vi "参数.vi"() -> ()   [LabVIEW 2018]
panel:
  in  "LOG":bool
  in  "选项卡控件":T1(tab)
  in  "轮盘关到开终点":dbl=10.0 caption="操作力终点" format="%.2f"
  in  "轮盘关到开起点":dbl=10.0 caption="操作力起点" format="%.2f"
  in  "轮盘关到开锁起点":dbl=10.0 caption="锁止力起点" format="%.2f"
  in  "轮盘关到开锁终点":dbl=10.0 caption="锁止力终点" format="%.2f"
  in  "轮盘关到开锁系数+":sgl=10.0 caption="锁止力系数+" format="%.2f"
  in  "轮盘关到开锁系数x":sgl=10.0 caption="锁止力系数x" format="%.2f"
  in  "轮盘关到开锁上限":sgl=10.0 caption="锁止力上限" format="%.2f"
  in  "轮盘关到开锁下限":sgl=10.0 caption="锁止力下限" format="%.2f"
  in  "轮盘关到开系数":sgl=10.0 caption="操作力系数" format="%.2f"
  in  "轮盘关到开曲线点数":dbl=10.0 caption="曲线点数"
  in  "轮盘关到开上限":sgl=10.0 caption="操作力上限" format="%.2f"
  in  "轮盘关到开下限":sgl=10.0 caption="操作力下限" format="%.2f"
  in  "轮盘关到开Y轴上限":dbl=10.0 caption="Y轴上限" format="%.1f"
  in  "轮盘关到开Y轴下限":dbl=10.0 caption="Y轴下限" format="%.1f"
  in  "轮盘开到关终点":dbl=10.0 caption="操作力终点" format="%.2f"
  in  "轮盘开到关起点":dbl=10.0 caption="操作力起点" format="%.2f"
  in  "轮盘开到关锁起点":dbl=10.0 caption="锁止力起点" format="%.2f"
  in  "轮盘开到关锁终点":dbl=10.0 caption="锁止力终点" format="%.2f"
  in  "轮盘开到关锁系数+":sgl=10.0 caption="锁止力系数+" format="%.2f"
  in  "轮盘开到关锁系数x":sgl=10.0 caption="锁止力系数x" format="%.2f"
  in  "轮盘开到关锁上限":sgl=10.0 caption="锁止力上限" format="%.2f"
  in  "轮盘开到关锁下限":sgl=10.0 caption="锁止力下限" format="%.2f"
  in  "轮盘开到关系数":sgl=10.0 caption="操作力系数" format="%.2f"
  in  "轮盘开到关曲线点数":dbl=10.0 caption="曲线点数"
  in  "轮盘开到关上限":sgl=10.0 caption="操作力上限" format="%.2f"
  in  "轮盘开到关下限":sgl=10.0 caption="操作力下限" format="%.2f"
  in  "轮盘开到关Y轴上限":dbl=10.0 caption="Y轴上限" format="%.1f"
  in  "轮盘开到关Y轴下限":dbl=10.0 caption="Y轴下限" format="%.1f"
  in  "拨钮右到左终点":dbl=10.0 caption="操作力终点" format="%.2f"
  in  "拨钮右到左起点":dbl=10.0 caption="操作力起点" format="%.2f"
  in  "拨钮右到左系数":sgl=10.0 caption="操作力系数" format="%.2f"
  in  "拨钮右到左曲线点数":dbl=10.0 caption="曲线点数"
  in  "拨钮右到左上限":sgl=10.0 caption="操作力上限" format="%.2f"
  in  "拨钮右到左下限":sgl=10.0 caption="操作力下限" format="%.2f"
  in  "拨钮右到左Y轴上限":dbl=10.0 caption="Y轴上限" format="%.1f"
  in  "拨钮右到左Y轴下限":dbl=10.0 caption="Y轴下限" format="%.1f"
  in  "拨钮左到右终点":dbl=10.0 caption="操作力终点" format="%.2f"
  in  "拨钮左到右起点":dbl=10.0 caption="操作力起点" format="%.2f"
  in  "拨钮左到右系数":sgl=10.0 caption="操作力系数" format="%.2f"
  in  "拨钮左到右曲线点数":dbl=10.0 caption="曲线点数"
  in  "拨钮左到右上限":sgl=10.0 caption="操作力上限" format="%.2f"
  in  "拨钮左到右下限":sgl=10.0 caption="操作力下限" format="%.2f"
  in  "拨钮左到右Y轴上限":dbl=10.0 caption="Y轴上限" format="%.1f"
  in  "拨钮左到右Y轴下限":dbl=10.0 caption="Y轴下限" format="%.1f"
  in  "拨钮下到上终点":dbl=10.0 caption="操作力终点" format="%.2f"
  in  "拨钮下到上起点":dbl=10.0 caption="操作力起点" format="%.2f"
  in  "拨钮下到上系数":sgl=10.0 caption="操作力系数" format="%.2f"
  in  "拨钮下到上曲线点数":dbl=10.0 caption="曲线点数"
  in  "拨钮下到上上限":sgl=10.0 caption="操作力上限" format="%.2f"
  in  "拨钮下到上下限":sgl=10.0 caption="操作力下限" format="%.2f"
  in  "拨钮下到上Y轴上限":dbl=10.0 caption="Y轴上限" format="%.1f"
  in  "拨钮下到上Y轴下限":dbl=10.0 caption="Y轴下限" format="%.1f"
  in  "拨钮上到下终点":dbl=10.0 caption="操作力终点" format="%.2f"
  in  "拨钮上到下起点":dbl=10.0 caption="操作力起点" format="%.2f"
  in  "拨钮上到下系数":sgl=10.0 caption="操作力系数" format="%.2f"
  in  "拨钮上到下曲线点数":dbl=10.0 caption="曲线点数"
  in  "拨钮上到下上限":sgl=10.0 caption="操作力上限" format="%.2f"
  in  "拨钮上到下下限":sgl=10.0 caption="操作力下限" format="%.2f"
  in  "拨钮上到下Y轴上限":dbl=10.0 caption="Y轴上限" format="%.1f"
  in  "拨钮上到下Y轴下限":dbl=10.0 caption="Y轴下限" format="%.1f"
  in  "伺服速度":sgl caption="N" format="%.1f"
  in  "气压稳定时间":sgl caption="N" format="%.1f"
  in  "LED电流下限":sgl caption="N" format="%.2f"
  in  "LED电流上限":sgl caption="N" format="%.2f"
  in  "风门开电压下限":sgl caption="N" format="%.2f"
  in  "风门开电压上限":sgl caption="N" format="%.2f"
  in  "风门闭电压下限":sgl caption="N" format="%.2f"
  in  "风门闭电压上限":sgl caption="N" format="%.2f"
  in  "压力下限":sgl caption="N" format="%.1f"
  in  "压力上限":sgl caption="N" format="%.1f"
  in  "泄漏量上限":sgl caption="N" format="%.2f"
  out "有值改变":bool
  in  "停止":bool
  in  "轮盘预压力":sgl caption="N" format="%.1f"
  # "参数设置"
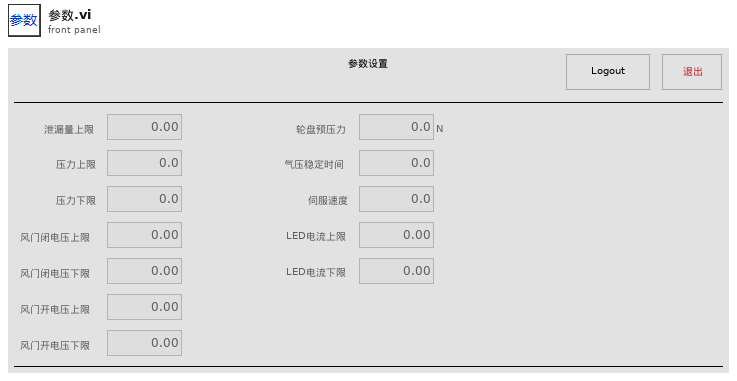
[diagram p1: front panel]
types:
  T1 = enum32{"轮盘关到开", "轮盘开到关", "拨钮右到左", "拨钮左到右", "拨钮下到上", "拨钮上到下"}
  T2 = enum8{"Enabled", "Disabled", "Disabled and Grayed Out"}
  T3 = cluster{"轮盘预压力":sgl, "泄漏量上限":sgl, "压力上限":sgl, "压力下限":sgl, "风门闭电压上限":sgl, "风门闭电压下限":sgl, "风门开电压上限":sgl, "风门开电压下限":sgl, "LED电流上限":sgl, "LED电流下限":sgl, "气压稳定时间":sgl, "伺服速度":sgl}
  T4 = cluster{"选择":enum16{"Fx", "Fy", "Fz", "Mx", "My", "Mz"}, "系数":sgl, "上限":sgl, "下限":sgl, "Ymax":dbl, "Ymin":dbl, "点数":dbl, "锁系数x":sgl, "锁上限":sgl, "锁下限":sgl, "锁系数+":sgl, "起点":dbl, "终点":dbl, "锁起点":dbl, "锁终点":dbl}
  T5 = cluster{"选择":enum16{"Fx", "Fy", "Fz", "Mx", "My", "Mz"}, "系数":sgl, "上限":sgl, "下限":sgl, "Ymax":dbl, "Ymin":dbl, "点数":dbl, "起点":dbl, "终点":dbl}
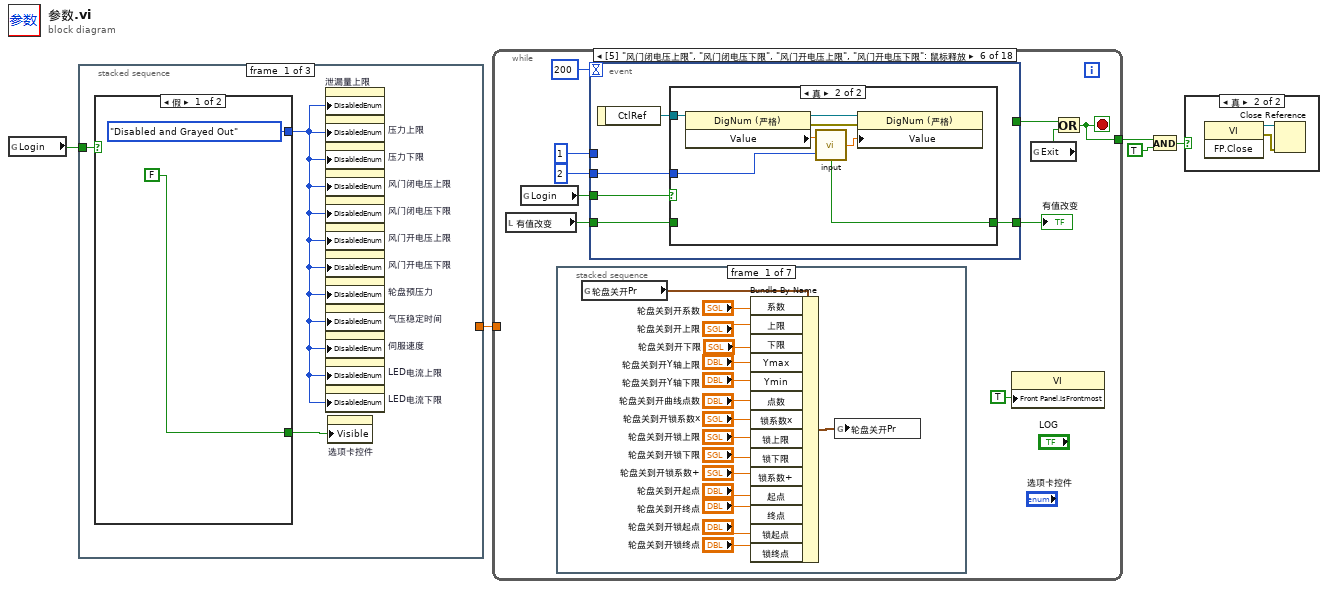
[diagram p0: block diagram]
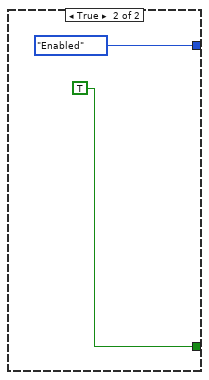
[diagram p2: hidden frame]
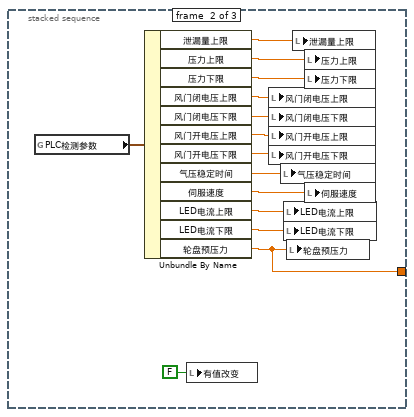
[diagram p3: hidden frame]
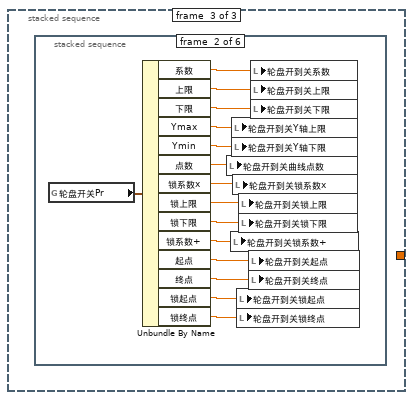
[diagram p4: hidden frame]
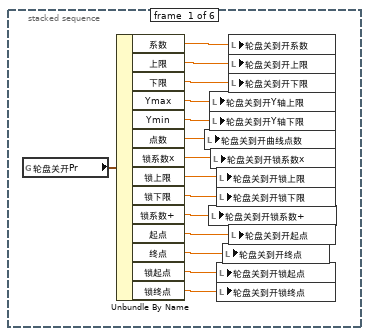
[diagram p5: hidden frame]
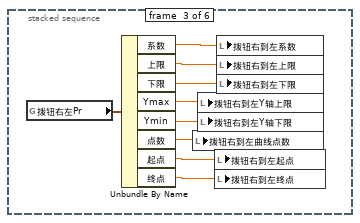
[diagram p6: hidden frame]
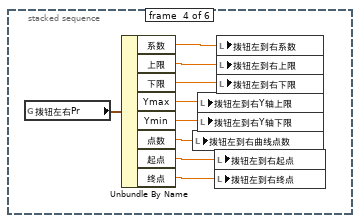
[diagram p7: hidden frame]
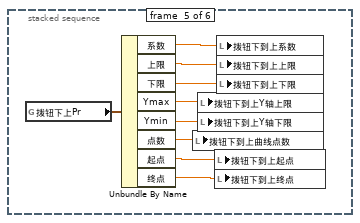
[diagram p8: hidden frame]
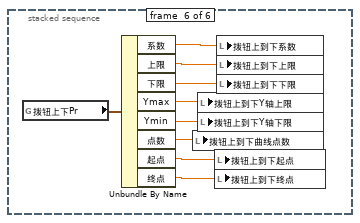
[diagram p9: hidden frame]
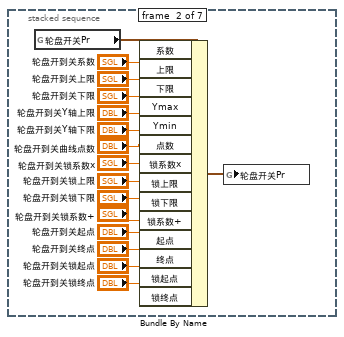
[diagram p11: hidden frame]
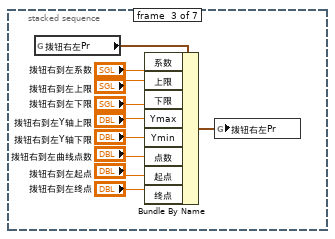
[diagram p12: hidden frame]
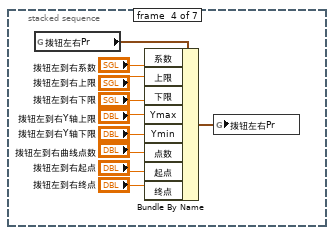
[diagram p13: hidden frame]
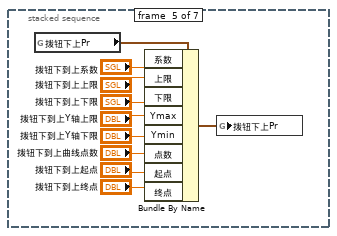
[diagram p14: hidden frame]
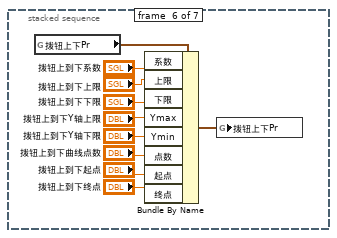
[diagram p15: hidden frame]
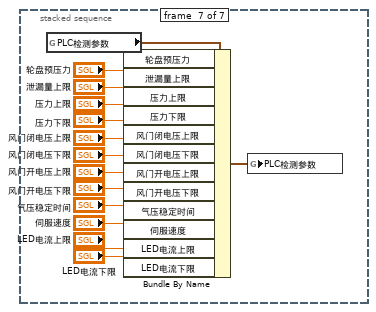
[diagram p16: hidden frame]
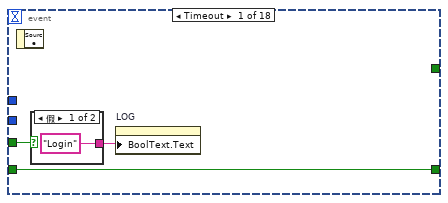
[diagram p17: hidden frame]
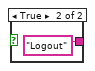
[diagram p18: hidden frame]
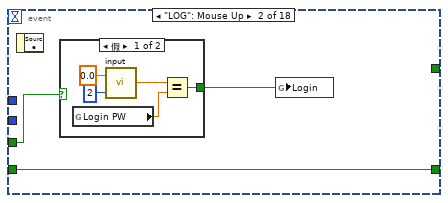
[diagram p19: hidden frame]
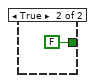
[diagram p20: hidden frame]
diagram:
  n1 = global read "全局 1.vi" "Login"() -> (w1:bool)
  n2 = stacked-sequence {
    tunnel: [_ w13 _] -> w2
    tunnel: w1 -> [w7 _ _]
    frame #0 {
      n3 = case shown="假" w7 {
        tunnel: [T2."Disabled and Grayed Out" ("禁用") T2."Enabled" ("禁用")] -> w8
        tunnel: [FALSE ("可见") TRUE ("可见")] -> w6
        frame False {
        }
        frame True {
        }
      }
      n4 = property on="泄漏量上限" class="DigNum (严格)"("DisabledEnum"=w8) -> ()  [unwired: 2 in, 2 out]
      n5 = property on="压力上限" class="DigNum (严格)"("DisabledEnum"=w8) -> ()  [unwired: 2 in, 2 out]
      n6 = property on="压力下限" class="DigNum (严格)"("DisabledEnum"=w8) -> ()  [unwired: 2 in, 2 out]
      n7 = property on="风门闭电压上限" class="DigNum (严格)"("DisabledEnum"=w8) -> ()  [unwired: 2 in, 2 out]
      n8 = property on="风门闭电压下限" class="DigNum (严格)"("DisabledEnum"=w8) -> ()  [unwired: 2 in, 2 out]
      n9 = property on="风门开电压上限" class="DigNum (严格)"("DisabledEnum"=w8) -> ()  [unwired: 2 in, 2 out]
      n10 = property on="风门开电压下限" class="DigNum (严格)"("DisabledEnum"=w8) -> ()  [unwired: 2 in, 2 out]
      n11 = property on="轮盘预压力" class="DigNum (严格)"("DisabledEnum"=w8) -> ()  [unwired: 2 in, 2 out]
      n12 = property on="气压稳定时间" class="DigNum (严格)"("DisabledEnum"=w8) -> ()  [unwired: 2 in, 2 out]
      n13 = property on="伺服速度" class="DigNum (严格)"("DisabledEnum"=w8) -> ()  [unwired: 2 in, 2 out]
      n14 = property on="LED电流上限" class="DigNum (严格)"("DisabledEnum"=w8) -> ()  [unwired: 2 in, 2 out]
      n15 = property on="LED电流下限" class="DigNum (严格)"("DisabledEnum"=w8) -> ()  [unwired: 2 in, 2 out]
      n16 = property on="选项卡控件" class="TabCtl (严格)"("Visible"=w6) -> ()  [unwired: 2 in, 2 out]
    }
    frame #1 {
      n17 = global read "全局 1.vi" "PLC检测参数"() -> (w15:T3)
      n18 = Unbundle By Name(w15) -> ("泄漏量上限"=w26:sgl, "压力上限"=w25:sgl, "压力下限"=w24:sgl, "风门闭电压上限"=w23:sgl, "风门闭电压下限"=w22:sgl, "风门开电压上限"=w21:sgl, "风门开电压下限"=w20:sgl, "气压稳定时间"=w19:sgl, "伺服速度"=w18:sgl, "LED电流上限"=w17:sgl, "LED电流下限"=w16:sgl, "轮盘预压力"=w13:sgl)
      n19 = local write "有值改变"(FALSE ("有值改变")) -> ()
      n20 = local write "风门闭电压上限"(w23) -> ()
      n21 = local write "风门闭电压下限"(w22) -> ()
      n22 = local write "风门开电压上限"(w21) -> ()
      n23 = local write "风门开电压下限"(w20) -> ()
      n24 = local write "气压稳定时间"(w19) -> ()
      n25 = local write "LED电流上限"(w17) -> ()
      n26 = local write "LED电流下限"(w16) -> ()
      n27 = local write "轮盘预压力"(w13) -> ()
      n28 = local write "泄漏量上限"(w26) -> ()
      n29 = local write "压力上限"(w25) -> ()
      n30 = local write "压力下限"(w24) -> ()
      n31 = local write "伺服速度"(w18) -> ()
    }
    frame #2 {
      n32 = stacked-sequence {
        frame #0 {
          n33 = global read "全局 1.vi" "轮盘关开Pr"() -> (w41:T4)
          n34 = Unbundle By Name(w41) -> ("系数"=w40:sgl, "上限"=w38:sgl, "下限"=w37:sgl, "Ymax"=w36:dbl, "Ymin"=w35:dbl, "点数"=w39:dbl, "锁系数x"=w32:sgl, "锁上限"=w34:sgl, "锁下限"=w33:sgl, "锁系数+"=w31:sgl, "起点"=w30:dbl, "终点"=w29:dbl, "锁起点"=w28:dbl, "锁终点"=w27:dbl)
          n35 = local write "轮盘关到开曲线点数"(w39) -> ()
          n36 = local write "轮盘关到开锁系数+"(w31) -> ()
          n37 = local write "轮盘关到开Y轴上限"(w36) -> ()
          n38 = local write "轮盘关到开Y轴下限"(w35) -> ()
          n39 = local write "轮盘关到开锁系数x"(w32) -> ()
          n40 = local write "轮盘关到开锁上限"(w34) -> ()
          n41 = local write "轮盘关到开锁下限"(w33) -> ()
          n42 = local write "轮盘关到开锁起点"(w28) -> ()
          n43 = local write "轮盘关到开锁终点"(w27) -> ()
          n44 = local write "轮盘关到开终点"(w29) -> ()
          n45 = local write "轮盘关到开系数"(w40) -> ()
          n46 = local write "轮盘关到开上限"(w38) -> ()
          n47 = local write "轮盘关到开下限"(w37) -> ()
          n48 = local write "轮盘关到开起点"(w30) -> ()
        }
        frame #1 {
          n49 = global read "全局 1.vi" "轮盘开关Pr"() -> (w56:T4)
          n50 = Unbundle By Name(w56) -> ("系数"=w55:sgl, "上限"=w53:sgl, "下限"=w52:sgl, "Ymax"=w51:dbl, "Ymin"=w50:dbl, "点数"=w54:dbl, "锁系数x"=w49:sgl, "锁上限"=w48:sgl, "锁下限"=w47:sgl, "锁系数+"=w46:sgl, "起点"=w45:dbl, "终点"=w44:dbl, "锁起点"=w43:dbl, "锁终点"=w42:dbl)
          n51 = local write "轮盘开到关曲线点数"(w54) -> ()
          n52 = local write "轮盘开到关锁系数+"(w46) -> ()
          n53 = local write "轮盘开到关Y轴上限"(w51) -> ()
          n54 = local write "轮盘开到关Y轴下限"(w50) -> ()
          n55 = local write "轮盘开到关锁系数x"(w49) -> ()
          n56 = local write "轮盘开到关锁起点"(w43) -> ()
          n57 = local write "轮盘开到关锁终点"(w42) -> ()
          n58 = local write "轮盘开到关锁上限"(w48) -> ()
          n59 = local write "轮盘开到关锁下限"(w47) -> ()
          n60 = local write "轮盘开到关起点"(w45) -> ()
          n61 = local write "轮盘开到关终点"(w44) -> ()
          n62 = local write "轮盘开到关系数"(w55) -> ()
          n63 = local write "轮盘开到关上限"(w53) -> ()
          n64 = local write "轮盘开到关下限"(w52) -> ()
        }
        frame #2 {
          n65 = global read "全局 1.vi" "拨钮右左Pr"() -> (w65:T5)
          n66 = Unbundle By Name(w65) -> ("系数"=w64:sgl, "上限"=w62:sgl, "下限"=w61:sgl, "Ymax"=w60:dbl, "Ymin"=w59:dbl, "点数"=w63:dbl, "起点"=w58:dbl, "终点"=w57:dbl)
          n67 = local write "拨钮右到左曲线点数"(w63) -> ()
          n68 = local write "拨钮右到左Y轴上限"(w60) -> ()
          n69 = local write "拨钮右到左Y轴下限"(w59) -> ()
          n70 = local write "拨钮右到左起点"(w58) -> ()
          n71 = local write "拨钮右到左终点"(w57) -> ()
          n72 = local write "拨钮右到左系数"(w64) -> ()
          n73 = local write "拨钮右到左上限"(w62) -> ()
          n74 = local write "拨钮右到左下限"(w61) -> ()
        }
        frame #3 {
          n75 = global read "全局 1.vi" "拨钮左右Pr"() -> (w74:T5)
          n76 = Unbundle By Name(w74) -> ("系数"=w73:sgl, "上限"=w71:sgl, "下限"=w70:sgl, "Ymax"=w69:dbl, "Ymin"=w68:dbl, "点数"=w72:dbl, "起点"=w67:dbl, "终点"=w66:dbl)
          n77 = local write "拨钮左到右曲线点数"(w72) -> ()
          n78 = local write "拨钮左到右Y轴上限"(w69) -> ()
          n79 = local write "拨钮左到右Y轴下限"(w68) -> ()
          n80 = local write "拨钮左到右起点"(w67) -> ()
          n81 = local write "拨钮左到右终点"(w66) -> ()
          n82 = local write "拨钮左到右系数"(w73) -> ()
          n83 = local write "拨钮左到右上限"(w71) -> ()
          n84 = local write "拨钮左到右下限"(w70) -> ()
        }
        frame #4 {
          n85 = global read "全局 1.vi" "拨钮下上Pr"() -> (w83:T5)
          n86 = Unbundle By Name(w83) -> ("系数"=w82:sgl, "上限"=w80:sgl, "下限"=w79:sgl, "Ymax"=w78:dbl, "Ymin"=w77:dbl, "点数"=w81:dbl, "起点"=w76:dbl, "终点"=w75:dbl)
          n87 = local write "拨钮下到上曲线点数"(w81) -> ()
          n88 = local write "拨钮下到上Y轴上限"(w78) -> ()
          n89 = local write "拨钮下到上Y轴下限"(w77) -> ()
          n90 = local write "拨钮下到上起点"(w76) -> ()
          n91 = local write "拨钮下到上终点"(w75) -> ()
          n92 = local write "拨钮下到上系数"(w82) -> ()
          n93 = local write "拨钮下到上上限"(w80) -> ()
          n94 = local write "拨钮下到上下限"(w79) -> ()
        }
        frame #5 {
          n95 = global read "全局 1.vi" "拨钮上下Pr"() -> (w92:T5)
          n96 = Unbundle By Name(w92) -> ("系数"=w91:sgl, "上限"=w89:sgl, "下限"=w88:sgl, "Ymax"=w87:dbl, "Ymin"=w86:dbl, "点数"=w90:dbl, "起点"=w84:dbl, "终点"=w85:dbl)
          n97 = local write "拨钮上到下曲线点数"(w90) -> ()
          n98 = local write "拨钮上到下Y轴上限"(w87) -> ()
          n99 = local write "拨钮上到下Y轴下限"(w86) -> ()
          n100 = local write "拨钮上到下起点"(w84) -> ()
          n101 = local write "拨钮上到下终点"(w85) -> ()
          n102 = local write "拨钮上到下系数"(w91) -> ()
          n103 = local write "拨钮上到下上限"(w89) -> ()
          n104 = local write "拨钮上到下下限"(w88) -> ()
        }
      }
    }
  }
  n105 = while {
    tunnel: [w99] -> w4
    tunnel: w2 -> [_]
    stop <- w99 stop-if-true
    n106 = local read "有值改变"() -> (w93:bool)
    n107 = global read "全局 1.vi" "Login"() -> (w94:bool)
    n108 = stacked-sequence {
      frame #0 {
        n109 = global read "全局 1.vi" "轮盘关开Pr"() -> (w104:T4)
        n110 = Bundle By Name(cluster=w104, "系数"="轮盘关到开系数", "上限"="轮盘关到开上限", "下限"="轮盘关到开下限", "Ymax"="轮盘关到开Y轴上限", "Ymin"="轮盘关到开Y轴下限", "点数"="轮盘关到开曲线点数", "锁系数x"="轮盘关到开锁系数x", "锁上限"="轮盘关到开锁上限", "锁下限"="轮盘关到开锁下限", "锁系数+"="轮盘关到开锁系数+", "起点"="轮盘关到开起点", "终点"="轮盘关到开终点", "锁起点"="轮盘关到开锁起点", "锁终点"="轮盘关到开锁终点") -> (w103:T4)
        n111 = global write "全局 1.vi" "轮盘关开Pr"(w103) -> ()
      }
      frame #1 {
        n112 = global read "全局 1.vi" "轮盘开关Pr"() -> (w134:T4)
        n113 = Bundle By Name(cluster=w134, "系数"="轮盘开到关系数", "上限"="轮盘开到关上限", "下限"="轮盘开到关下限", "Ymax"="轮盘开到关Y轴上限", "Ymin"="轮盘开到关Y轴下限", "点数"="轮盘开到关曲线点数", "锁系数x"="轮盘开到关锁系数x", "锁上限"="轮盘开到关锁上限", "锁下限"="轮盘开到关锁下限", "锁系数+"="轮盘开到关锁系数+", "起点"="轮盘开到关起点", "终点"="轮盘开到关终点", "锁起点"="轮盘开到关锁起点", "锁终点"="轮盘开到关锁终点") -> (w133:T4)
        n114 = global write "全局 1.vi" "轮盘开关Pr"(w133) -> ()
      }
      frame #2 {
        n115 = global read "全局 1.vi" "拨钮右左Pr"() -> (w144:T5)
        n116 = Bundle By Name(cluster=w144, "系数"="拨钮右到左系数", "上限"="拨钮右到左上限", "下限"="拨钮右到左下限", "Ymax"="拨钮右到左Y轴上限", "Ymin"="拨钮右到左Y轴下限", "点数"="拨钮右到左曲线点数", "起点"="拨钮右到左起点", "终点"="拨钮右到左终点") -> (w143:T5)
        n117 = global write "全局 1.vi" "拨钮右左Pr"(w143) -> ()
      }
      frame #3 {
        n118 = global read "全局 1.vi" "拨钮左右Pr"() -> (w154:T5)
        n119 = Bundle By Name(cluster=w154, "系数"="拨钮左到右系数", "上限"="拨钮左到右上限", "下限"="拨钮左到右下限", "Ymax"="拨钮左到右Y轴上限", "Ymin"="拨钮左到右Y轴下限", "点数"="拨钮左到右曲线点数", "起点"="拨钮左到右起点", "终点"="拨钮左到右终点") -> (w153:T5)
        n120 = global write "全局 1.vi" "拨钮左右Pr"(w153) -> ()
      }
      frame #4 {
        n121 = global read "全局 1.vi" "拨钮下上Pr"() -> (w164:T5)
        n122 = Bundle By Name(cluster=w164, "系数"="拨钮下到上系数", "上限"="拨钮下到上上限", "下限"="拨钮下到上下限", "Ymax"="拨钮下到上Y轴上限", "Ymin"="拨钮下到上Y轴下限", "点数"="拨钮下到上曲线点数", "起点"="拨钮下到上起点", "终点"="拨钮下到上终点") -> (w163:T5)
        n123 = global write "全局 1.vi" "拨钮下上Pr"(w163) -> ()
      }
      frame #5 {
        n124 = global read "全局 1.vi" "拨钮上下Pr"() -> (w174:T5)
        n125 = Bundle By Name(cluster=w174, "系数"="拨钮上到下系数", "上限"="拨钮上到下上限", "下限"="拨钮上到下下限", "Ymax"="拨钮上到下Y轴上限", "Ymin"="拨钮上到下Y轴下限", "点数"="拨钮上到下曲线点数", "起点"="拨钮上到下起点", "终点"="拨钮上到下终点") -> (w173:T5)
        n126 = global write "全局 1.vi" "拨钮上下Pr"(w173) -> ()
      }
      frame #6 {
        n127 = global read "全局 1.vi" "PLC检测参数"() -> (w175:T3)
        n128 = Bundle By Name(cluster=w175, "轮盘预压力"="轮盘预压力", "泄漏量上限"="泄漏量上限", "压力上限"="压力上限", "压力下限"="压力下限", "风门闭电压上限"="风门闭电压上限", "风门闭电压下限"="风门闭电压下限", "风门开电压上限"="风门开电压上限", "风门开电压下限"="风门开电压下限", "气压稳定时间"="气压稳定时间", "伺服速度"="伺服速度", "LED电流上限"="LED电流上限", "LED电流下限"="LED电流下限") -> (w188:T3)
        n129 = global write "全局 1.vi" "PLC检测参数"(w188) -> ()
      }
    }
    n130 = event shown="[5] \"风门闭电压上限\", \"风门闭电压下限\", \"风门开电压上限\", \"风门开电压下限\": 鼠标释放" {
      selector: _ -> [_ _ _ _ _ _ _ _ _ _ _ _ _ _ _ _ _ _]
      dyn-events: _ -> [_ _ _ _ _ _ _ _ _ _ _ _ _ _ _ _ _ _]
      timeout: 200 -> [_ _ _ _ _ _ _ _ _ _ _ _ _ _ _ _ _ _]
      tunnel: [_ _ "停止" _ _ _ _ _ _ _ _ _ _ _ _ _ _ _] -> w98
      tunnel: 1 -> [_ _ _ _ w223 _ _ w262 w275 w288 _ _ _ _ _ w334 w341 _]
      tunnel: 2 -> [_ _ _ w210 _ w236 w246 _ _ _ w298 w307 w314 w321 w328 _ _ _]
      tunnel: [w189 w194 w203 w207 w222 w235 w249 w261 w274 w287 w300 w306 w313 w320 w327 w335 w342 w349] -> w95
      tunnel: w94 -> [w191 w195 _ w209 w220 w234 w248 w260 w273 w286 _ _ _ _ _ _ _ _]
      tunnel: w93 -> [w189 w194 w203 w208 w221 w233 w247 w259 w272 w285 _ _ _ _ _ _ _ _]
      event Timeout {
        n131 = event-data() -> ()  [unwired: 1 in, 1 out]
        n132 = case shown="假" w191 {
          tunnel: ["Login" "Logout"] -> w190
          frame False {
          }
          frame True {
          }
        }
        n133 = property on="LOG" class="Bool"("BoolText.Text"=w190) -> ()  [unwired: 2 in, 2 out]
      }
      event "LOG": Mouse Up {
        n134 = event-data() -> ()  [unwired: 1 in, 1 out]
        n135 = case shown="假" w195 {
          tunnel: [w197 FALSE] -> w196
          frame False {
            n136 = global read "全局 1.vi" "Login PW"() -> (w198:dbl)
            n137 = call "input.vi"("位数(2)"=2, "in"=0.0) -> ("out"=w199:dbl)  [unwired: 1 out]
            n138 = Equal?(x=w199, y=w198) -> (x = y?=w197:bool)
          }
          frame True {
          }
        }
        n139 = global write "全局 1.vi" "Login"(w196) -> ()
      }
      event "停止": Value Change {
        n140 = event-data() -> ()  [unwired: 1 in, 1 out]
        n141 = global read "全局 1.vi" "ini文件"() -> (w204:path)
        n142 = case shown="真" w203 {
          tunnel: w204 -> [_ w206]
          frame False {
          }
          frame True {
            n143 = call "WriteIni.vi"("configuration file path"=w206) -> ()  [unwired: 1 in]
          }
        }
      }
      event "泄漏量上限": Mouse Up {
        n144 = event-data() -> ("CtlRef"=w211:refnum<vi>)  [unwired: 1 in]
        n145 = case shown="假" w209 {
          tunnel: w211 -> [_ w219]
          tunnel: w210 -> [_ w217]
          tunnel: w208 -> [w212 _]
          tunnel: [w212 w213] -> w207
          frame False {
          }
          frame True {
            n146 = property class="DigNum (严格)"(reference=w219) -> (reference out=w216:refnum<vi>, error out=w215:errorcluster, "Value"=w218:sgl)  [unwired: 1 in]
            n147 = call "input.vi"("位数(2)"=w217, "in"=w218) -> ("out"=w214:dbl, "值改变?"=w213:bool)
            n148 = property class="DigNum (严格)"(reference=w216, error in=w215, "Value"=w214) -> ()  [unwired: 2 out]
          }
        }
      }
      event "压力上限", "压力下限": Mouse Up {
        n149 = event-data() -> ("CtlRef"=w224:refnum<vi>)  [unwired: 1 in]
        n150 = case shown="真" w220 {
          tunnel: w224 -> [_ w232]
          tunnel: w223 -> [_ w230]
          tunnel: [w225 w229] -> w222
          tunnel: w221 -> [w225 _]
          frame False {
          }
          frame True {
            n151 = property class="DigNum (严格)"(reference=w232) -> (reference out=w228:refnum<vi>, error out=w227:errorcluster, "Value"=w231:sgl)  [unwired: 1 in]
            n152 = call "input.vi"("位数(2)"=w230, "in"=w231) -> ("out"=w226:dbl, "值改变?"=w229:bool)
            n153 = property class="DigNum (严格)"(reference=w228, error in=w227, "Value"=w226) -> ()  [unwired: 2 out]
          }
        }
      }
      event "风门闭电压上限", "风门闭电压下限", "风门开电压上限", "风门开电压下限": Mouse Up {
        n154 = event-data() -> ("CtlRef"=w237:refnum<vi>)  [unwired: 1 in]
        n155 = case shown="真" w234 {
          tunnel: w237 -> [_ w245]
          tunnel: w236 -> [_ w243]
          tunnel: [w238 w242] -> w235
          tunnel: w233 -> [w238 _]
          frame False {
          }
          frame True {
            n156 = property class="DigNum (严格)"(reference=w245) -> (reference out=w241:refnum<vi>, error out=w240:errorcluster, "Value"=w244:sgl)  [unwired: 1 in]
            n157 = call "input.vi"("位数(2)"=w243, "in"=w244) -> ("out"=w239:dbl, "值改变?"=w242:bool)
            n158 = property class="DigNum (严格)"(reference=w241, error in=w240, "Value"=w239) -> ()  [unwired: 2 out]
          }
        }
      }
      event "LED电流上限", "LED电流下限": Mouse Up {
        n159 = event-data() -> ("CtlRef"=w250:refnum<vi>)  [unwired: 1 in]
        n160 = case shown="真" w248 {
          tunnel: w250 -> [_ w258]
          tunnel: w246 -> [_ w256]
          tunnel: [w251 w255] -> w249
          tunnel: w247 -> [w251 _]
          frame False {
          }
          frame True {
            n161 = property class="DigNum (严格)"(reference=w258) -> (reference out=w254:refnum<vi>, error out=w253:errorcluster, "Value"=w257:sgl)  [unwired: 1 in]
            n162 = call "input.vi"("位数(2)"=w256, "in"=w257) -> ("out"=w252:dbl, "值改变?"=w255:bool)
            n163 = property class="DigNum (严格)"(reference=w254, error in=w253, "Value"=w252) -> ()  [unwired: 2 out]
          }
        }
      }
      event "气压稳定时间": Mouse Up {
        n164 = event-data() -> ("CtlRef"=w263:refnum<vi>)  [unwired: 1 in]
        n165 = case shown="真" w260 {
          tunnel: w263 -> [_ w271]
          tunnel: w262 -> [_ w269]
          tunnel: [w264 w268] -> w261
          tunnel: w259 -> [w264 _]
          frame False {
          }
          frame True {
            n166 = property class="DigNum (严格)"(reference=w271) -> (reference out=w267:refnum<vi>, error out=w266:errorcluster, "Value"=w270:sgl)  [unwired: 1 in]
            n167 = call "input.vi"("位数(2)"=w269, "in"=w270) -> ("out"=w265:dbl, "值改变?"=w268:bool)
            n168 = property class="DigNum (严格)"(reference=w267, error in=w266, "Value"=w265) -> ()  [unwired: 2 out]
          }
        }
      }
      event "伺服速度": Mouse Up {
        n169 = event-data() -> ("CtlRef"=w276:refnum<vi>)  [unwired: 1 in]
        n170 = case shown="假" w273 {
          tunnel: w276 -> [_ w284]
          tunnel: w275 -> [_ w282]
          tunnel: [w277 w281] -> w274
          tunnel: w272 -> [w277 _]
          frame False {
          }
          frame True {
            n171 = property class="DigNum (严格)"(reference=w284) -> (reference out=w279:refnum<vi>, error out=w278:errorcluster, "Value"=w283:sgl)  [unwired: 1 in]
            n172 = call "input.vi"("位数(2)"=w282, "in"=w283) -> ("out"=w280:dbl, "值改变?"=w281:bool)
            n173 = property class="DigNum (严格)"(reference=w279, error in=w278, "Value"=w280) -> ()  [unwired: 2 out]
          }
        }
      }
      event "轮盘预压力": Mouse Up {
        n174 = event-data() -> ("CtlRef"=w289:refnum<vi>)  [unwired: 1 in]
        n175 = case shown="真" w286 {
          tunnel: w289 -> [_ w297]
          tunnel: w288 -> [_ w295]
          tunnel: [w290 w294] -> w287
          tunnel: w285 -> [w290 _]
          frame False {
          }
          frame True {
            n176 = property class="DigNum (严格)"(reference=w297) -> (reference out=w293:refnum<vi>, error out=w292:errorcluster, "Value"=w296:sgl)  [unwired: 1 in]
            n177 = call "input.vi"("位数(2)"=w295, "in"=w296) -> ("out"=w291:dbl, "值改变?"=w294:bool)
            n178 = property class="DigNum (严格)"(reference=w293, error in=w292, "Value"=w291) -> ()  [unwired: 2 out]
          }
        }
      }
      event "拨钮上到下系数", "拨钮下到上系数", "拨钮左到右系数", "拨钮右到左系数", "轮盘开到关系数", "轮盘关到开系数", "轮盘关到开锁系数x", "轮盘开到关锁系数x", "轮盘关到开锁系数+", "轮盘开到关锁系数+": Mouse Up {
        n179 = event-data() -> ("CtlRef"=w304:refnum<vi>)  [unwired: 1 in]
        n180 = property class="DigNum (严格)"(reference=w304) -> (reference out=w302:refnum<vi>, error out=w299:errorcluster, "Value"=w303:sgl)  [unwired: 1 in]
        n181 = call "input.vi"("位数(2)"=w298, "in"=w303) -> ("out"=w301:dbl, "值改变?"=w300:bool)
        n182 = property class="DigNum (严格)"(reference=w302, error in=w299, "Value"=w301) -> ()  [unwired: 2 out]
      }
      event "拨钮上到下上限", "拨钮下到上上限", "拨钮左到右上限", "拨钮右到左上限", "轮盘开到关上限", "轮盘关到开上限", "轮盘关到开锁上限", "轮盘开到关锁上限": Mouse Up {
        n183 = event-data() -> ("CtlRef"=w311:refnum<vi>)  [unwired: 1 in]
        n184 = property class="DigNum (严格)"(reference=w311) -> (reference out=w309:refnum<vi>, error out=w305:errorcluster, "Value"=w310:sgl)  [unwired: 1 in]
        n185 = call "input.vi"("位数(2)"=w307, "in"=w310) -> ("out"=w308:dbl, "值改变?"=w306:bool)
        n186 = property class="DigNum (严格)"(reference=w309, error in=w305, "Value"=w308) -> ()  [unwired: 2 out]
      }
      event "拨钮上到下下限", "拨钮下到上下限", "拨钮左到右下限", "拨钮右到左下限", "轮盘开到关下限", "轮盘关到开下限", "轮盘关到开锁下限", "轮盘开到关锁下限": Mouse Up {
        n187 = event-data() -> ("CtlRef"=w318:refnum<vi>)  [unwired: 1 in]
        n188 = property class="DigNum (严格)"(reference=w318) -> (reference out=w316:refnum<vi>, error out=w312:errorcluster, "Value"=w317:sgl)  [unwired: 1 in]
        n189 = call "input.vi"("位数(2)"=w314, "in"=w317) -> ("out"=w315:dbl, "值改变?"=w313:bool)
        n190 = property class="DigNum (严格)"(reference=w316, error in=w312, "Value"=w315) -> ()  [unwired: 2 out]
      }
      event "轮盘关到开锁起点", "轮盘开到关锁起点", "轮盘开到关起点", "轮盘关到开起点", "拨钮右到左起点", "拨钮左到右起点", "拨钮上到下起点", "拨钮下到上起点": Mouse Up {
        n191 = event-data() -> ("CtlRef"=w325:refnum<vi>)  [unwired: 1 in]
        n192 = property class="DigNum (严格)"(reference=w325) -> (reference out=w323:refnum<vi>, error out=w319:errorcluster, "Value"=w324:dbl)  [unwired: 1 in]
        n193 = call "input.vi"("位数(2)"=w321, "in"=w324) -> ("out"=w322:dbl, "值改变?"=w320:bool)
        n194 = property class="DigNum (严格)"(reference=w323, error in=w319, "Value"=w322) -> ()  [unwired: 2 out]
      }
      event "轮盘关到开锁终点", "轮盘开到关锁终点", "轮盘关到开终点", "轮盘开到关终点", "拨钮右到左终点", "拨钮左到右终点", "拨钮下到上终点", "拨钮上到下终点": Mouse Up {
        n195 = event-data() -> ("CtlRef"=w332:refnum<vi>)  [unwired: 1 in]
        n196 = property class="DigNum (严格)"(reference=w332) -> (reference out=w330:refnum<vi>, error out=w326:errorcluster, "Value"=w331:dbl)  [unwired: 1 in]
        n197 = call "input.vi"("位数(2)"=w328, "in"=w331) -> ("out"=w329:dbl, "值改变?"=w327:bool)
        n198 = property class="DigNum (严格)"(reference=w330, error in=w326, "Value"=w329) -> ()  [unwired: 2 out]
      }
      event "拨钮上到下Y轴上限", "拨钮下到上Y轴上限", "拨钮左到右Y轴上限", "拨钮右到左Y轴上限", "轮盘开到关Y轴上限", "轮盘关到开Y轴上限": Mouse Up {
        n199 = event-data() -> ("CtlRef"=w339:refnum<vi>)  [unwired: 1 in]
        n200 = property class="DigNum (严格)"(reference=w339) -> (reference out=w337:refnum<vi>, error out=w333:errorcluster, "Value"=w338:dbl)  [unwired: 1 in]
        n201 = call "input.vi"("位数(2)"=w334, "in"=w338) -> ("out"=w336:dbl, "值改变?"=w335:bool)
        n202 = property class="DigNum (严格)"(reference=w337, error in=w333, "Value"=w336) -> ()  [unwired: 2 out]
      }
      event "拨钮上到下Y轴下限", "拨钮下到上Y轴下限", "拨钮左到右Y轴下限", "拨钮右到左Y轴下限", "轮盘开到关Y轴下限", "轮盘关到开Y轴下限": Mouse Up {
        n203 = event-data() -> ("CtlRef"=w346:refnum<vi>)  [unwired: 1 in]
        n204 = property class="DigNum (严格)"(reference=w346) -> (reference out=w344:refnum<vi>, error out=w340:errorcluster, "Value"=w345:dbl)  [unwired: 1 in]
        n205 = call "input.vi"("位数(2)"=w341, "in"=w345) -> ("out"=w343:dbl, "值改变?"=w342:bool)
        n206 = property class="DigNum (严格)"(reference=w344, error in=w340, "Value"=w343) -> ()  [unwired: 2 out]
      }
      event "拨钮上到下曲线点数", "拨钮下到上曲线点数", "拨钮左到右曲线点数", "拨钮右到左曲线点数", "轮盘开到关曲线点数", "轮盘关到开曲线点数": Mouse Up {
        n207 = event-data() -> ("CtlRef"=w353:refnum<vi>)  [unwired: 1 in]
        n208 = property class="DigNum (严格)"(reference=w353) -> (reference out=w351:refnum<vi>, error out=w347:errorcluster, "Value"=w352:dbl)  [unwired: 1 in]
        n209 = call "input.vi"("位数(2)"=0, "in"=w352) -> ("out"=w350:dbl, "值改变?"=w349:bool)
        n210 = property class="DigNum (严格)"(reference=w351, error in=w347, "Value"=w350) -> ()  [unwired: 2 out]
      }
    }
    "有值改变" <- w95
    n211 = property class="VI"("Front Panel.IsFrontmost"=TRUE ("前面板窗口:在最前")) -> ()  [unwired: 2 in, 2 out]
    n212 = global read "全局 1.vi" "Exit"() -> (w97:bool)
    n213 = Or(x=w98, y=w97) -> (x .or. y?=w99:bool)
  }
  n214 = And(x=w4, y=TRUE) -> (x .and. y?=w5:bool)
  n215 = case shown="真" w5 {
    frame False {
    }
    frame True {
      n216 = invoke class="VI" method="FP.Close"() -> (reference out=w354:refnum<vi>, error out=w355:errorcluster)  [unwired: 3 in, 1 out]
      n217 = Close Reference(reference=w354, error in (no error)=w355) -> ()  [unwired: 1 out]
    }
  }
